vi "rd_lbne.vi"(1 "ADDRESS 2":i16) -> (0 "DATA 2":u32 format="%x")   [LabVIEW 2014]
doc: "This VI is designed to be used with the UDP Receiver VI. Run the UDP Receiver.vi first.\n\nThe UDP protocol differs from TCP in that there is no error-checking with the packets of information that are sent, and thus no guarantee whatsoever that an intended recipient will actually receive a given piece of data.\n\nUDP does offer the ability to \"broadcast\" data across a network--simply specify an IP Address of all ones (255.255.255.255) to attempt to broadcast information network-wide. Keep in mind that routers and other network hardware will generally refuse to forward the broadcast beyond certain points, so the extent of the broadcast will in practice be limited."
uses:
  LBNE_Global .vi
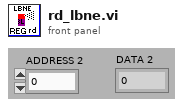
[diagram p1: front panel]
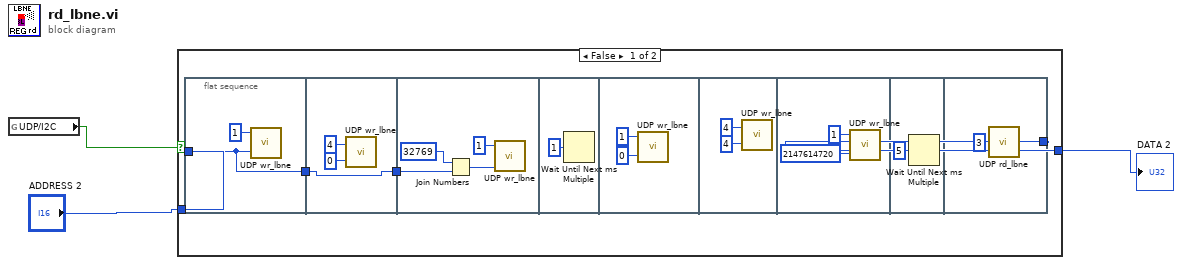
[diagram p0: block diagram]
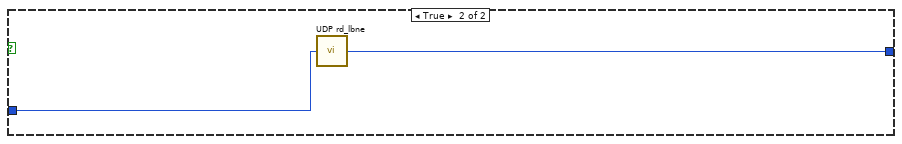
[diagram p2: hidden frame]
diagram:
  n1 = global read "LBNE_Global .vi" "UDP/I2C"() -> (w3:bool)
  n2 = case shown="False" w3 {
    tunnel: "ADDRESS 2" -> [w5 w28]
    tunnel: [w4 w27] -> w2
    frame False {
      n3 = flat-sequence {
        tunnel: w5 -> [w8]
        tunnel: [w8] -> w7
        tunnel: w7 -> [w10]
        tunnel: [w10] -> w6
        tunnel: w6 -> [w14]
        tunnel: [w25] -> w4
        frame #0 {
          n4 = call "UDP wr_lbne.vi"("DATA"=w8, "ADDRESS"=u16 1) -> ()  [unwired: 1 out]
        }
        frame #1 {
          n5 = call "UDP wr_lbne.vi"("DATA"=u32 0, "ADDRESS"=u16 4) -> ()  [unwired: 1 out]
        }
        frame #2 {
          n6 = Join Numbers(hi=u16 32769, lo=w14) -> ((hi.lo)=w15:u32)
          n7 = call "UDP wr_lbne.vi"("DATA"=w15, "ADDRESS"=u16 1) -> ()  [unwired: 1 out]
        }
        frame #3 {
          n8 = Wait Until Next ms Multiple(millisecond multiple=u32 1) -> ()  [unwired: 1 out]
        }
        frame #4 {
          n9 = call "UDP wr_lbne.vi"("DATA"=u32 0, "ADDRESS"=u16 1) -> ()  [unwired: 1 out]
        }
        frame #5 {
          n10 = call "UDP wr_lbne.vi"("DATA"=u32 4, "ADDRESS"=u16 4) -> ()  [unwired: 1 out]
        }
        frame #6 {
          n11 = call "UDP wr_lbne.vi"("DATA"=u32 2147614720, "ADDRESS"=u16 1) -> ()  [unwired: 1 out]
        }
        frame #7 {
          n12 = Wait Until Next ms Multiple(millisecond multiple=u32 5) -> ()  [unwired: 1 out]
        }
        frame #8 {
          n13 = call "UDP rd_lbne.vi"("ADDRESS 2"=i16 3) -> ("DATA 2"=w25:u32)
        }
      }
    }
    frame True {
      n14 = call "UDP rd_lbne.vi"("ADDRESS 2"=w28) -> ("DATA 2"=w27:u32)
    }
  }
  "DATA 2" <- w2
